vi "UI - Initiate Connection.vi"(8 "error in (no error)":errorcluster, 10 "Controller Address":string, 11 "Message Queue":refnum<queue>) -> (0 "error out":errorcluster, 1 "Connected?":bool)   [LabVIEW 2018]
uses:
  Message Queue/Message Cluster.ctl
  controls/Control State.ctl
  controls/Variable References.ctl
  controls/IO References.ctl
  Globals/Global - Configuration Options.vi
  Globals/Global - UI Stream and Variable Connections.vi
  Message Queue/Message Queue.lvlib
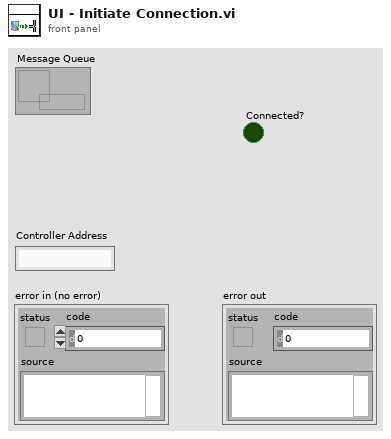
[diagram p1: front panel]
types:
  T1 = typedef "Control State.ctl" = enum16{"Safe State", "Control (PID)"}
  T2 = typedef "Message Queue.lvlib/Message Cluster.ctl" = cluster{"Message":string, "Message Data":variant}
  T3 = typedef "IO References.ctl" = cluster{"Control Input Values":refnum<k21>[], "Control Output Values":refnum<k21>[], "Temperature Values":refnum<k21>[], "Threshold Exceeded":refnum<k21>}
  T4 = typedef "Variable References.ctl" = cluster{"CPU Usage":refnum<k21>, "Contiguous Memory":refnum<k21>, "Control Mode":refnum<k21>, "Control Loop Period":refnum<k21>, "Low Speed Loop Period":refnum<k21>}
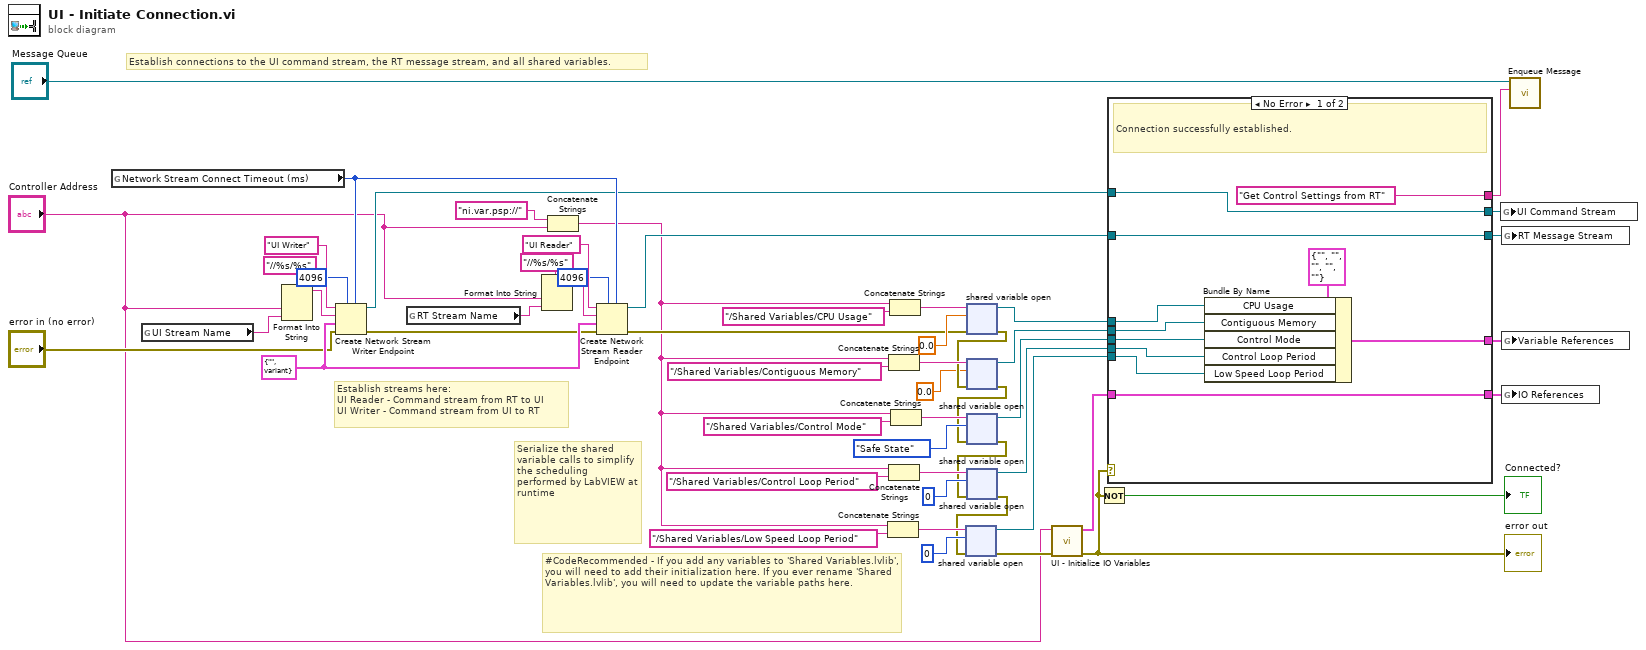
[diagram p0: block diagram]
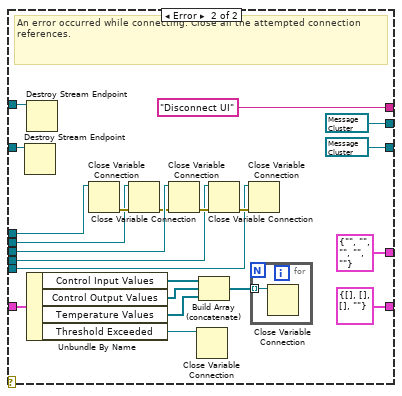
[diagram p2: hidden frame]
diagram:
  w45 = T2 {"Message"="", "Message Data"=variant} ("Message Cluster")
  # "Establish connections to the UI command stream, the RT message stream, and all shared variables."
  # "#CodeRecommended - If you add any variables to 'Shared Variables.lvlib', you will need to add their initialization here. If you ever rename 'Shared Variables.lvlib', you will need to update the variable paths here."
  # "Establish streams here:\nUI Reader - Command stream from RT to UI\nUI Writer - Command stream from UI to RT"
  # "Serialize the shared variable calls to simplify the scheduling performed by LabVIEW at runtime"
  n1 = global read "Global - Configuration Options.vi" "Network Stream Connect Timeout (ms)"() -> (w44:i32)
  n2 = global read "Global - Configuration Options.vi" "UI Stream Name"() -> (w52:string)
  n3 = Format Into String(format string="//%s/%s", "Controller Address", w52) -> (resulting string=w51:string)  [unwired: 2 in, 1 out]
  n4 = Create Network Stream Writer Endpoint(5:w44, 7:4096 ("writer buffer size"), 8:"error in (no error)", 9:w45, 10:w51, 11:"UI Writer" ("writer name")) -> (0:w17:errorcluster, 3:w25:refnum<k21>)  [unwired: 1 in]
  n5 = global read "Global - Configuration Options.vi" "RT Stream Name"() -> (w49:string)
  n6 = Format Into String(format string="//%s/%s", "Controller Address", w49) -> (resulting string=w48:string)  [unwired: 2 in, 1 out]
  n7 = Concatenate Strings("ni.var.psp://", "Controller Address") -> (w10:string)
  n8 = Create Network Stream Reader Endpoint(5:w44, 7:4096 ("reader buffer size"), 8:w17, 9:w45, 10:w48, 11:"UI Reader" ("reader name")) -> (0:w16:errorcluster, 3:w24:refnum<k21>)  [unwired: 1 in]
  n9 = Concatenate Strings(w10, "/Shared Variables/Low Speed Loop Period") -> (w14:string)
  n10 = Concatenate Strings(w10, "/Shared Variables/Contiguous Memory") -> (w38:string)
  n11 = Concatenate Strings(w10, "/Shared Variables/Control Loop Period") -> (w34:string)
  n12 = Concatenate Strings(w10, "/Shared Variables/CPU Usage") -> (w41:string)
  n13 = Concatenate Strings(w10, "/Shared Variables/Control Mode") -> (w37:string)
  n14 = shared-variable-open(w41, w16, 0.0) -> (w29:refnum<k21>, w31:errorcluster)  [unwired: 1 in]
  n15 = shared-variable-open(w38, w31, 0.0) -> (w28:refnum<k21>, w9:errorcluster)  [unwired: 1 in]
  n16 = shared-variable-open(w37, w9, Control_State."Safe State" ("FPGA State")) -> (w27:refnum<k21>, w30:errorcluster)  [unwired: 1 in]
  n17 = shared-variable-open(w34, w30, u32 0) -> (w26:refnum<k21>, w13:errorcluster)  [unwired: 1 in]
  n18 = shared-variable-open(w14, w13, u32 0) -> (w12:refnum<k21>, w7:errorcluster)  [unwired: 1 in]
  n19 = call "UI - Initialize IO Variables.vi"("error in (no error)"=w7, "Controller Address"="Controller Address") -> ("error out"=w6:errorcluster, "IO References"=w4:T3)  [unwired: 8 in]
  "error out" <- w6
  n20 = Not(x=w6) -> (.not. x?=→"Connected?":bool)
  n21 = case shown="No Error" w6 {
    tunnel: w29 -> [w64 w83]
    tunnel: w28 -> [w63 w80]
    tunnel: w27 -> [w62 w81]
    tunnel: w26 -> [w61 w82]
    tunnel: w25 -> [w57 w86]
    tunnel: w24 -> [w59 w87]
    tunnel: [w60 T4 {"CPU Usage"="", "Contiguous Memory"="", "Control Mode"="", "Control Loop Period"="", "Low Speed Loop Period"=""} ("Variable References")] -> w23
    tunnel: [w59 refnum<k21> refnum] -> w22
    tunnel: [w57 refnum<k21> refnum] -> w21
    tunnel: ["Get Control Settings from RT" "Disconnect UI"] -> w19
    tunnel: w12 -> [w56 w74]
    tunnel: [w55 T3 {"Control Input Values"=[], "Control Output Values"=[], "Temperature Values"=[], "Threshold Exceeded"=""} ("IO References")] -> w8
    tunnel: w4 -> [w55 w71]
    frame No Error {
      # "Connection successfully established."
      n22 = Bundle By Name(cluster=T4 {"CPU Usage"="", "Contiguous Memory"="", "Control Mode"="", "Control Loop Period"="", "Low Speed Loop Period"=""} ("Variable References"), "CPU Usage"=w64, "Contiguous Memory"=w63, "Control Mode"=w62, "Control Loop Period"=w61, "Low Speed Loop Period"=w56) -> (w60:T4)
    }
    frame Error {
      # "An error occurred while connecting. Close all the attempted connection references."
      n23 = Destroy Stream Endpoint(11:w87) -> ()  [unwired: 1 in, 1 out]
      n24 = Destroy Stream Endpoint(11:w86) -> ()  [unwired: 1 in, 1 out]
      n25 = Unbundle By Name(w71) -> ("Control Input Values"=w70:refnum<k21>[], "Control Output Values"=w69:refnum<k21>[], "Temperature Values"=w68:refnum<k21>[], "Threshold Exceeded"=w66:refnum<k21>)
      n26 = Close Variable Connection(11:w83) -> (0:w84:errorcluster)  [unwired: 1 in]
      n27 = Close Variable Connection(8:w84, 11:w80) -> (0:w73:errorcluster)
      n28 = Close Variable Connection(8:w73, 11:w81) -> (0:w85:errorcluster)
      n29 = Close Variable Connection(11:w66) -> ()  [unwired: 1 in, 1 out]
      n30 = Build Array (concatenate)(w70, w69, w68) -> (w67:refnum<k21>[])
      n31 = Close Variable Connection(8:w85, 11:w82) -> (0:w75:errorcluster)
      n32 = Close Variable Connection(8:w75, 11:w74) -> ()  [unwired: 1 out]
      n33 = for {
        tunnel: w67 -> [w88] mode=indexing
        n34 = Close Variable Connection(11:w88) -> ()  [unwired: 1 in, 1 out]
      }
    }
  }
  n35 = global write "Global - UI Stream and Variable Connections.vi" "UI Command Stream"(w21) -> ()
  n36 = global write "Global - UI Stream and Variable Connections.vi" "RT Message Stream"(w22) -> ()
  n37 = global write "Global - UI Stream and Variable Connections.vi" "Variable References"(w23) -> ()
  n38 = global write "Global - UI Stream and Variable Connections.vi" "IO References"(w8) -> ()
  n39 = call "Enqueue Message.vi"("Message"=w19, "Message Queue"="Message Queue") -> ()  [unwired: 8 in, 2 out]
